vi "PXIe-433x Main Page.vi"(8 "error in (no error)":errorcluster, 11 "Node Ptr":T3 format="%.0x") -> (0 "error out":errorcluster)   [LabVIEW 2011, in "PXIe-433x Custom Device.lvlib"]
uses:
  PXIe-433x Custom Device.lvlib
  <vilib>/NI Veristand/Custom Device API/Custom Device Item Ref.ctl
  <vilib>/NI Veristand/Custom Device API/Custom Device Timed Loop Priority.ctl
  Mode.ctl
  <vilib>/NI Veristand/Custom Device API/Custom Device Execution Mode.ctl
  <vilib>/NI Veristand/Custom Device API/Path Specification.ctl
  <vilib>/NI Veristand/Custom Device API/Path Type.ctl
  Global.vi
  <vilib>/NI Veristand/Custom Device API/Get Item Property (U16).vi
  <vilib>/NI Veristand/Custom Device API/Get Item Property (Double).vi
  <vilib>/NI Veristand/Custom Device API/Get Item Property (I32).vi
  <vilib>/NI Veristand/Custom Device API/Set Item Property (I32).vi
  <vilib>/NI Veristand/Custom Device API/Set Item Property (Double).vi
  <vilib>/NI Veristand/Custom Device API/Set Item Property (U16).vi
  <vilib>/NI Veristand/Custom Device API/Custom Device API.lvlib
panel:
  in  "String (transparent)":string="If there is no other timing master in the system (DAQ, FPGA, etc) then you must set this device as the master on the controller and chassis pages."
  in  "Mode":T1
  in  "Hardware Rate":dbl
  in  "Priority":T2
  in  "Core Assignment":i32
  in  "Header":cluster{"Section Name":string}={"Section Name"="PXIe-4330 or 4331 Devices"}
  in  "Description":string
  in  "Custom Device Name":string
  # "(-2 is automatic)"
  # "(-2 is max)"
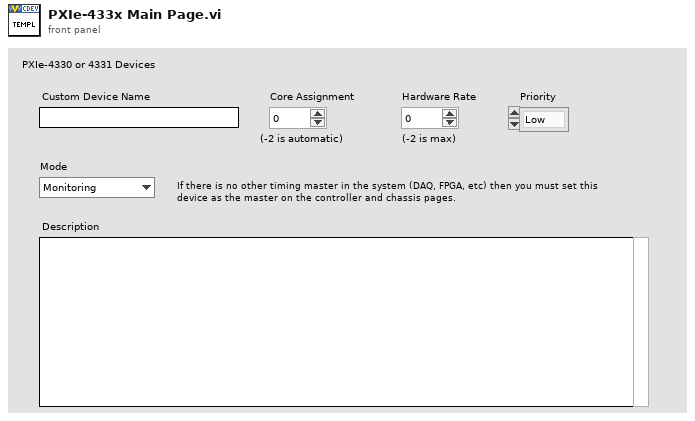
[diagram p1: front panel]
types:
  T1 = typedef "PXIe-433x Custom Device.lvlib/Mode.ctl" = enum16{"Monitoring", "Control"}
  T2 = typedef "Custom Device API.lvlib/Custom Device Timed Loop Priority.ctl" = enum32{"Low", "Medium", "High"}
  T3 = typedef "Custom Device API.lvlib/Custom Device Item Ref.ctl" = u64
  T4 = typedef "Custom Device API.lvlib/Custom Device Item Info.ctl" = cluster{"Name":string, "Is Channel":bool, "GUID":string}
  T5 = enum8{"Enabled", "Disabled", "Disabled and Grayed Out"}
  T6 = typedef "Custom Device API.lvlib/Custom Device Execution Mode.ctl" = enum16{"Asynchronous", "Inline HW Interface", "Inline Model Interface", "Inline Timing and Sync", "Asynchronous Timing and Sync"}
  T7 = typedef "Custom Device API.lvlib/Path Specification.ctl" = cluster{"Path":path, "Type":T8}
  T8 = typedef "Custom Device API.lvlib/Path Type.ctl" = enum16{"Absolute", "To Base", "To Common Data Dir", "To Application Data Dir"}
  T9 = cluster{"Execution mode":T6, "Driver VI Path (RT)":path, "Driver VI Path (Host)":T7}[]
  T10 = typedef "Custom Device API.lvlib/Custom Device Commands.ctl" = enum16{"Default", "Item renamed", "Shutdown", "Dynamic button pressed"}
  T11 = cluster{"Execution mode":T6, "Driver VI Path (RT)":path, "Driver VI Path (Host)":T7}
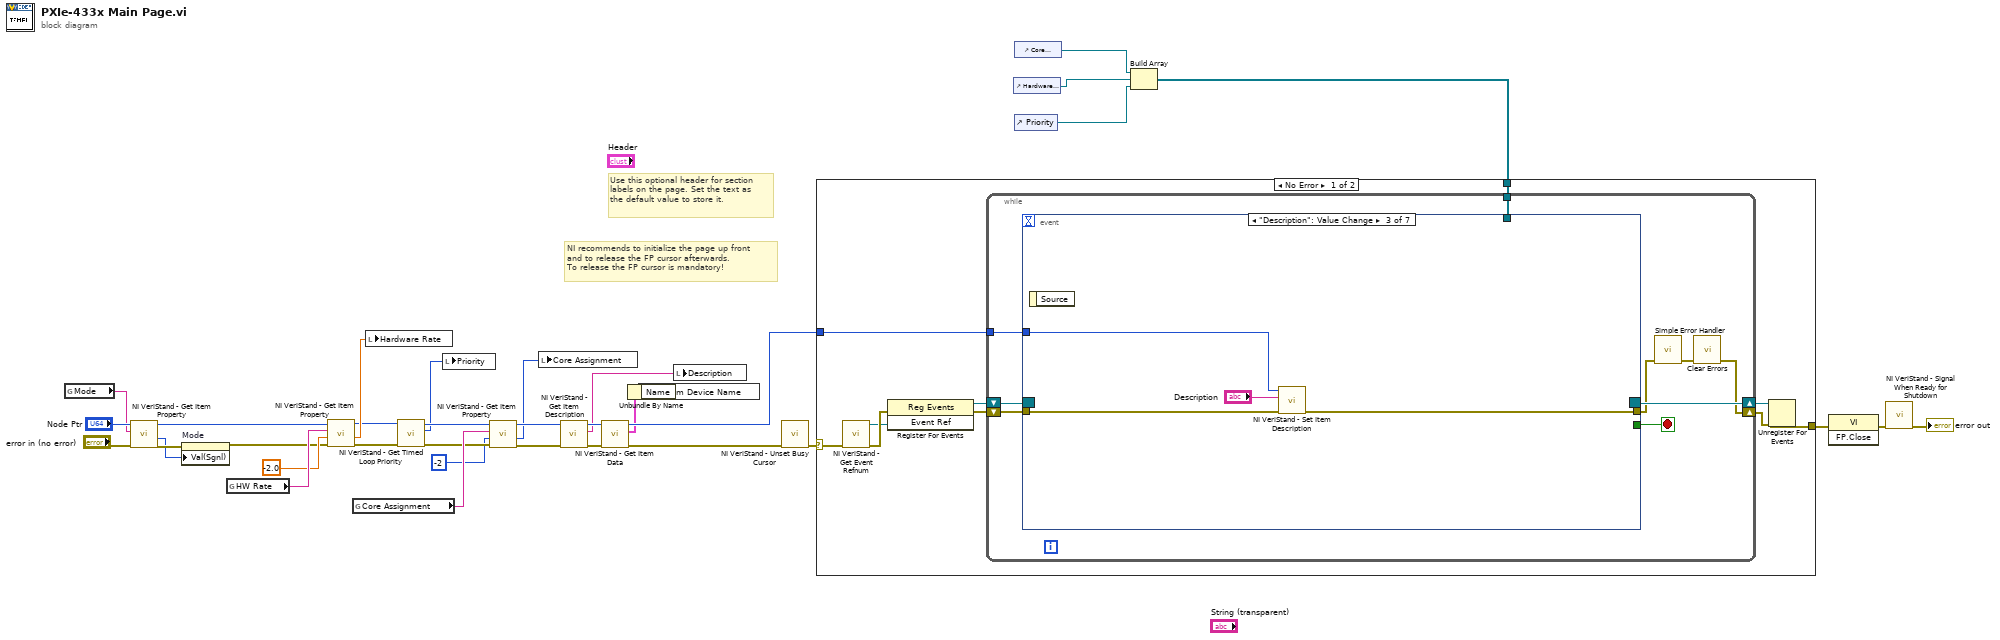
[diagram p0: block diagram]
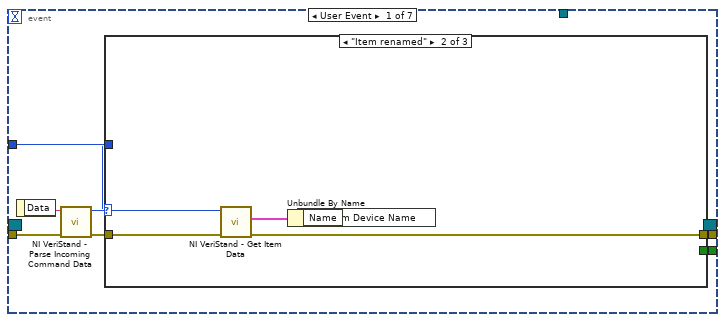
[diagram p2: hidden frame]
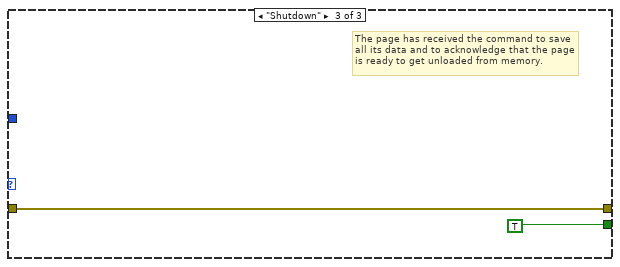
[diagram p4: hidden frame]
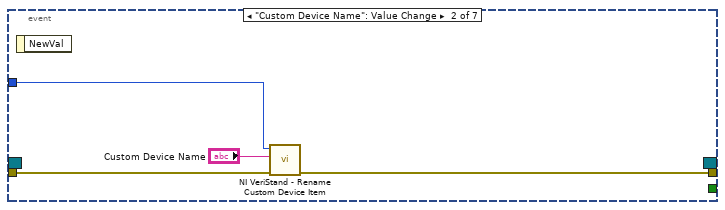
[diagram p5: hidden frame]
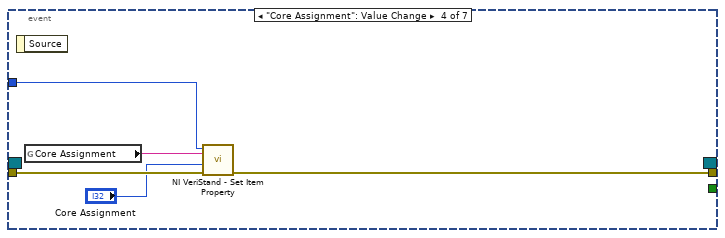
[diagram p6: hidden frame]
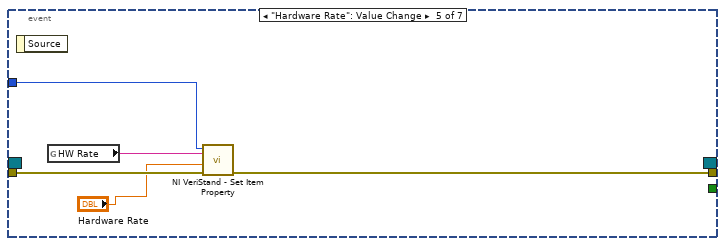
[diagram p7: hidden frame]
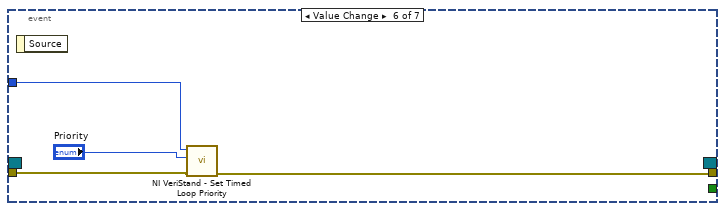
[diagram p8: hidden frame]
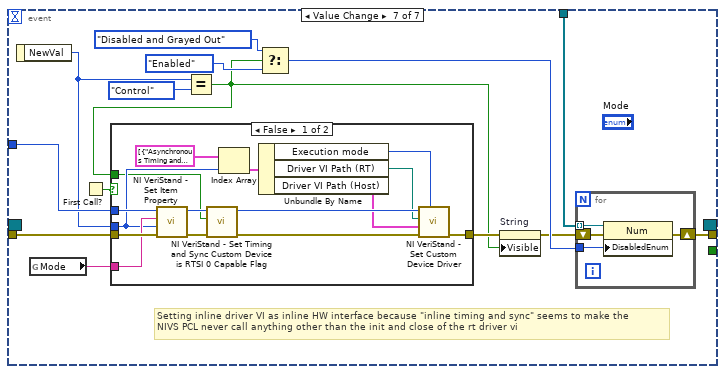
[diagram p9: hidden frame]
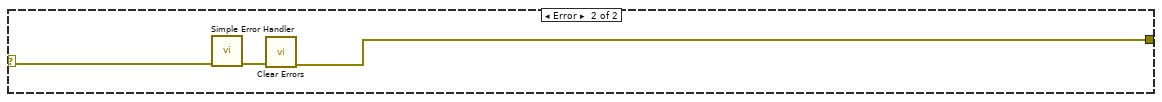
[diagram p11: hidden frame]
diagram:
  # "Use this optional header for section labels on the page. Set the text as the default value to store it."
  # "NI recommends to initialize the page up front\nand to release the FP cursor afterwards.\nTo release the FP cursor is mandatory!"
  n1 = global read "Global.vi" "Mode"() -> (w11:string)
  n2 = call-poly <vilib>:"NI VeriStand - Get Item Property.vi"("error in (no error)"="error in (no error)", "Property Name"=w11, "Item Ref in"="Node Ptr") -> ("error out"=w10:errorcluster, "Value"=w9:u16, "Item Ref out"=w8:T3)  [unwired: 5 in, 1 out]
  n3 = property on="Mode" class="Enum (strict)"(error in=w10, "Val(Sgnl)"=w9) -> (error out=w7:errorcluster)  [unwired: 1 in, 1 out]
  n4 = global read "Global.vi" "HW Rate"() -> (w17:string)
  n5 = call-poly <vilib>:"NI VeriStand - Get Item Property.vi"("error in (no error)"=w7, "Default Value"=-2.0, "Property Name"=w17, "Item Ref in"=w8) -> ("error out"=w13:errorcluster, "Value"=w15:dbl, "Item Ref out"=w14:T3)  [unwired: 4 in, 1 out]
  n6 = global read "Global.vi" "Core Assignment"() -> (w30:string)
  n7 = local write "Hardware Rate"(w15) -> ()
  n8 = call <vilib>:"NI VeriStand - Get Timed Loop Priority.vi"("error in (no error)"=w13, "Device Ref in"=w14) -> ("error out"=w24:errorcluster, "Priority"=w19:T2, "Device Ref out"=w22:T3)  [unwired: 7 in]
  n9 = local write "Priority"(w19) -> ()
  n10 = call-poly <vilib>:"NI VeriStand - Get Item Property.vi"("error in (no error)"=w24, "Default Value"=-2, "Property Name"=w30, "Item Ref in"=w22) -> ("error out"=w23:errorcluster, "Value"=w20:i32, "Item Ref out"=w21:T3)  [unwired: 4 in, 1 out]
  n11 = local write "Core Assignment"(w20) -> ()
  n12 = call <vilib>:"NI VeriStand - Get Item Description.vi"("error in (no error)"=w23, "Item Ref in"=w21) -> ("error out"=w27:errorcluster, "Description"=w28:string, "Item Ref out"=w29:T3)  [unwired: 7 out]
  n13 = call <vilib>:"NI VeriStand - Get Item Data.vi"("error in (no error)"=w27, "Item Ref in"=w29) -> ("error out"=w2:errorcluster, "Item Info"=w26:T4, "Item Ref out"=w31:T3)  [unwired: 7 out]
  n14 = Unbundle By Name(w26) -> ("Name"=w25:string)
  n15 = local write "Custom Device Name"(w25) -> ()
  n16 = local write "Description"(w28) -> ()
  n17 = call <vilib>:"NI VeriStand - Unset Busy Cursor.vi"("error in (no error)"=w2) -> ("error out"=w32:errorcluster)  [unwired: 10 out]
  n18 = control-ref of="Hardware Rate"() -> (w5:refnum<vi>)
  n19 = control-ref of="Core Assignment"() -> (w4:refnum<vi>)
  n20 = control-ref of="Priority"() -> (w6:refnum<vi>)
  n21 = Build Array(w4, w5, w6) -> (w3:refnum<vi>[])
  n22 = case shown="No Error" w32 {
    selector: w32 -> [w37 w128]
    tunnel: [w42 w126] -> w35
    tunnel: w31 -> [w38 _]
    tunnel: w3 -> [w36 _]
    frame No Error {
      n23 = call <vilib>:"NI VeriStand - Get Event Refnum.vi"("error in (no error)"=w37) -> ("error out"=w45:errorcluster, "Event Ref"=w41:refnum<user-event>)  [unwired: 9 out]
      n24 = register-events(error in=w45, w41) -> (reference out=w39:refnum<event-registration>, error out=w40:errorcluster)  [unwired: 1 in]
      n25 = while {
        tunnel: w38 -> [w50]
        shift-right: [w47] -> w43
        shift-left: w40 -> [w53]
        shift-right: [w54] -> w44
        shift-left: w39 -> [w52]
        tunnel: w36 -> [w46]
        stop <- w51 stop-if-true
        n26 = event shown="[2] \"Description\": Value Change" {
          selector: w52 -> [_ _ _ _ _ _ _]
          dyn-events: [_ _ _ _ _ _ _] -> w54
          timeout: _ -> [_ _ _ _ _ _ _]
          tunnel: w53 -> [w61 w73 w76 w82 w87 w91 w103]
          tunnel: [w57 _ _ _ _ _ _] -> w51
          tunnel: [w56 w72 w75 w78 w84 w88 w104] -> w49
          tunnel: w50 -> [w55 w71 w77 w81 w86 w90 w102]
          tunnel: w46 -> [_ _ _ _ _ _ w105]
          event User Event {
            n27 = event-data() -> ("Data"=w60:string)  [unwired: 1 out]
            n28 = call <vilib>:"NI VeriStand - Parse Incoming Command Data.vi"("error in (no error)"=w61, "Incoming data"=w60) -> ("error out"=w59:errorcluster, "Action"=w58:T10)  [unwired: 8 out]
            n29 = case shown="\"Item renamed\"" w58 {
              tunnel: w59 -> [w62 w67 w68]
              tunnel: [_ _ TRUE] -> w57
              tunnel: [w62 w64 w68] -> w56
              tunnel: w55 -> [_ w66 _]
              frame "Default", Default {
              }
              frame "Item renamed" {
                n30 = call <vilib>:"NI VeriStand - Get Item Data.vi"("error in (no error)"=w67, "Item Ref in"=w66) -> ("error out"=w64:errorcluster, "Item Info"=w65:T4)  [unwired: 8 out]
                n31 = Unbundle By Name(w65) -> ("Name"=w63:string)
                n32 = local write "Custom Device Name"(w63) -> ()
              }
              frame "Shutdown" {
                # "The page has received the command to save all its data and to acknowledge that the page is ready to get unloaded from memory."
              }
            }
          }
          event "Custom Device Name": Value Change {
            n33 = event-data() -> ()  [unwired: 2 out]
            n34 = call <vilib>:"NI VeriStand - Rename Custom Device Item.vi"("error in (no error)"=w73, "New Name"="Custom Device Name", "Item Ref in"=w71) -> ("error out"=w72:errorcluster)  [unwired: 8 out]
          }
          event "Description": Value Change {
            n35 = event-data() -> ()  [unwired: 2 out]
            n36 = call <vilib>:"NI VeriStand - Set Item Description.vi"("error in (no error)"=w76, "Description"="Description", "Item Ref in"=w77) -> ("error out"=w75:errorcluster)  [unwired: 8 out]
          }
          event "Core Assignment": Value Change {
            n37 = event-data() -> ()  [unwired: 2 out]
            n38 = global read "Global.vi" "Core Assignment"() -> (w80:string)
            n39 = call-poly <vilib>:"NI VeriStand - Set Item Property.vi"("error in (no error)"=w82, "Value"="Core Assignment", "Property Name"=w80, "Item Ref in"=w81) -> ("error out"=w78:errorcluster)  [unwired: 5 in, 2 out]
          }
          event "Hardware Rate": Value Change {
            n40 = event-data() -> ()  [unwired: 2 out]
            n41 = global read "Global.vi" "HW Rate"() -> (w85:string)
            n42 = call-poly <vilib>:"NI VeriStand - Set Item Property.vi"("error in (no error)"=w87, "Value"="Hardware Rate", "Property Name"=w85, "Item Ref in"=w86) -> ("error out"=w84:errorcluster)  [unwired: 5 in, 2 out]
          }
          event Value Change {
            n43 = event-data() -> ()  [unwired: 2 out]
            n44 = call <vilib>:"NI VeriStand - Set Timed Loop Priority.vi"("error in (no error)"=w91, "Priority"="Priority", "Device Ref in"=w90) -> ("error out"=w88:errorcluster)  [unwired: 7 in, 1 out]
          }
          event Value Change {
            # "Setting inline driver VI as inline HW interface because \"inline timing and sync\" seems to make the\nNIVS PCL never call anything other than the init and close of the rt driver vi"
            n45 = event-data() -> ("NewVal"=w100:T1)  [unwired: 1 out]
            n46 = global read "Global.vi" "Mode"() -> (w95:string)
            n47 = First Call?() -> (First Call?: T/F=w101:bool)
            n48 = Equal?(x=w100, y=Mode."Control") -> (x = y?=w92:bool)
            n49 = case shown="False" w101 {
              tunnel: w103 -> [w120 w121]
              tunnel: [w107 w121] -> w94
              tunnel: w102 -> [w119 _]
              tunnel: w100 -> [w113 _]
              tunnel: w92 -> [w108 _]
              tunnel: w95 -> [w116 _]
              frame False {
                n50 = call-poly <vilib>:"NI VeriStand - Set Item Property.vi"("error in (no error)"=w120, "Value"=w113, "Property Name"=w116, "Item Ref in"=w119) -> ("error out"=w118:errorcluster, "Item Ref out"=w117:T3)  [unwired: 5 in, 1 out]
                n51 = call <vilib>:"NI VeriStand - Set Timing and Sync Custom Device is RTSI 0 Capable Flag.vi"("error in (no error)"=w118, "Is RTSI 0 Capable"=w108, "Device Ref in"=w117) -> ("error out"=w115:errorcluster, "Device Ref out"=w114:T3)  [unwired: 7 in]
                n52 = Index Array(array=T9 [{"Execution mode"=enum."Asynchronous Timing and Sync", "Driver VI Path (RT)"=path "c:/ni-rt/NIVeriStand2010/Timing and Sync/PXIe-433x/PXIe-433x RT Driver VI.vi", "Driver VI Path (Host)"={"Path"=path "Timing and Sync/PXIe-433x/PXIe-433x RT Driver VI.vi", "Type"=enum."To Common Data Dir"}}, {"Execution mode"=enum."Inline HW Interface", "Driver VI Path (RT)"=path "c:/ni-rt/NIVeriStand2010/Timing and Sync/PXIe-433x/PXIe-433x Inline RT Driver VI.vi", "Driver VI Path (Host)"={"Path"=path "Timing and Sync/PXIe-433x/PXIe-433x Inline RT Driver VI.vi", "Type"=enum."To Common Data Dir"}}], index=w113) -> (element=w112:T11)
                n53 = Unbundle By Name(w112) -> ("Execution mode"=w111:T6, "Driver VI Path (RT)"=w109:path, "Driver VI Path (Host)"=w110:T7)
                n54 = call <vilib>:"NI VeriStand - Set Custom Device Driver.vi"("Execution mode"=w111, "error in (no error)"=w115, "Driver VI Path (Host)"=w110, "Driver VI Path (RT)"=w109, "Device Ref in"=w114) -> ("error out"=w107:errorcluster)  [unwired: 5 in, 1 out]
              }
              frame True {
                # "Called by init, don't make any changes to avoid dirty dot"
              }
            }
            n55 = Select(t=T5."Disabled and Grayed Out" ("Disabled"), s=w92, f=T5."Enabled" ("Disabled")) -> (s? t:f=w96:T5)
            n56 = property on="String" class="Str"(error in=w94, "Visible"=w92) -> (error out=w93:errorcluster)  [unwired: 1 in, 1 out]
            n57 = for {
              tunnel: w96 -> [w124]
              tunnel: w105 -> [w123] mode=indexing
              shift-right: [w122] -> w104
              shift-left: w93 -> [w125]
              n58 = property on="Property Node" class="Num"(reference=w123, error in=w125, "DisabledEnum"=w124) -> (error out=w122:errorcluster)  [unwired: 1 out]
            }
          }
        }
        n59 = call <vilib>:"Simple Error Handler.vi"("error in (no error)"=w49) -> ("error out"=w48:errorcluster)  [unwired: 1 in, 7 out]
        n60 = call <vilib>:"Clear Errors.vi"("error in (no error)"=w48) -> ("error out"=w47:errorcluster)  [unwired: 6 out]
      }
      n61 = Unregister For Events(event registration refnum=w44, error in=w43) -> (error out=w42:errorcluster)
    }
    frame Error {
      n62 = call <vilib>:"Simple Error Handler.vi"("error in (no error)"=w128) -> ("error out"=w127:errorcluster)  [unwired: 1 in, 7 out]
      n63 = call <vilib>:"Clear Errors.vi"("error in (no error)"=w127) -> ("error out"=w126:errorcluster)  [unwired: 6 out]
    }
  }
  n64 = invoke class="VI" method="FP.Close"(error in=w35) -> (error out=w34:errorcluster)  [unwired: 2 in, 2 out]
  n65 = call <vilib>:"NI VeriStand - Signal When Ready for Shutdown.vi"("error in (no error)"=w34) -> ("error out"=→"error out":errorcluster)  [unwired: 10 out]
